vi "InspectCall.vi"(7 "ConcreteActor":refnum<class "ConcreteActor.lvclass">, 11 "Message":refnum<class "Message.lvclass">) -> (3 "Message":refnum<class "Message.lvclass">, 5 "ConcreteActor":refnum<class "ConcreteActor.lvclass">)   [LabVIEW 2020, in "_Template.lvlib" / "ActorTemplate.lvlib" / "{{Name}}.lvlib" / "ConcreteActor.lvclass"]
uses:
  ConcreteActor.lvclass
  jettl/jettl/Message/Message.lvclass
  ConcreteActor.lvclass/ConcreteActor.ctl
  jettl/jettl/Actor/Actor.lvclass
panel:
  # "This front panel should not be manipulated."
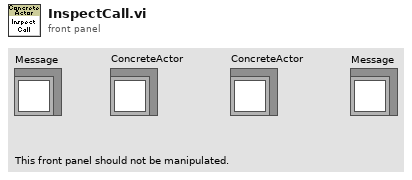
[diagram p1: front panel]
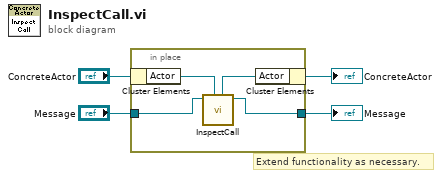
[diagram p0: block diagram]
diagram:
  # "Extend functionality as necessary."
  n1 = in-place {
    in-place-border: "Message" -> [w6]
    in-place-border: [w5] -> w1
    n2 = in-place-cluster #1("ConcreteActor") -> ("Actor"=w8:refnum<class "Actor.lvclass">)
    n3 = call-dynamic "InspectCall.vi"("Actor"=w8, "Message"=w6) -> ("Message"=w5:refnum<class "Message.lvclass">, "Actor"=w7:refnum<class "Actor.lvclass">)  [unwired: 8 in]
    n4 = in-place-cluster #1("Actor"=w7) -> (→"ConcreteActor":refnum<class "ConcreteActor.lvclass">)
  }
  "Message" <- w1
